vi "CRYASIO Receive Global Data.vi"(8 "buf count":i32=-1, 9 "Chn Idx":u32, 10 "Data Length":i32, 11 "Last Remain Buffer":i32[](array[numeric])) -> (0 "Over Load":i32, 1 "bufCount":i32, 2 "Data Out":i32[](array[numeric]), 3 "Remain Data":i32[](array[numeric]))   [LabVIEW 2013]
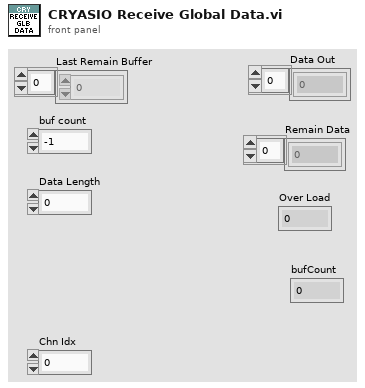
[diagram p1: front panel]
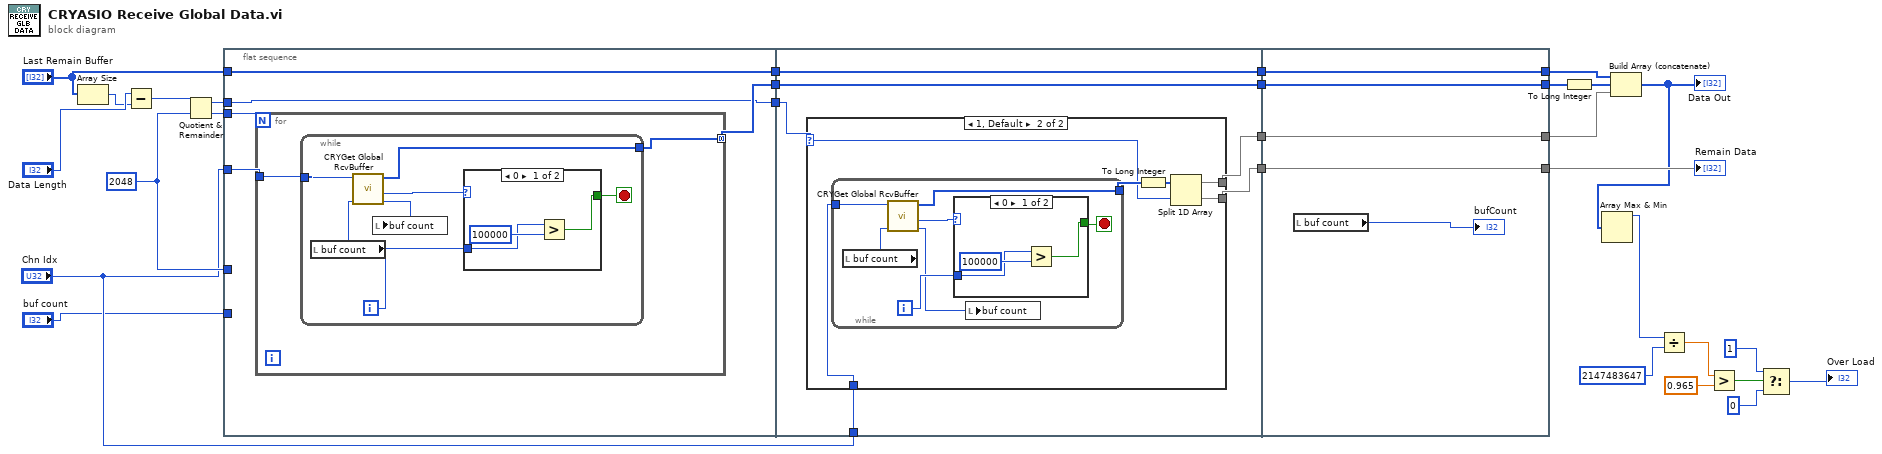
[diagram p0: block diagram]
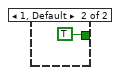
[diagram p2: hidden frame]
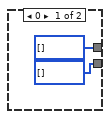
[diagram p3: hidden frame]
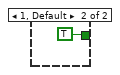
[diagram p4: hidden frame]
diagram:
  w30 = 2048 ("y")
  n1 = Array Size(array="Last Remain Buffer") -> (size(s)=w28:i32)
  n2 = Subtract(x="Data Length", y=w28) -> (x-y=w27:i32)
  n3 = Quotient & Remainder(x=w27, y=w30) -> (x-y*floor(x/y)=w19:i32, floor(x/y)=w26:i32)
  n4 = flat-sequence {
    tunnel: w30 -> [_]
    tunnel: w26 -> [w35]
    tunnel: [w34] -> w23
    tunnel: [w33] -> w22
    tunnel: "Last Remain Buffer" -> [w33]
    tunnel: w19 -> [w32]
    tunnel: [w32] -> w18
    tunnel: "Chn Idx" -> [w31]
    tunnel: "buf count" -> [_]
    tunnel: w23 -> [w54]
    tunnel: w22 -> [w53]
    tunnel: w18 -> [w52]
    tunnel: "Chn Idx" -> [w49]
    tunnel: [w54] -> w13
    tunnel: [w53] -> w12
    tunnel: [w51] -> w11
    tunnel: [w50] -> w10
    tunnel: [w75] -> w16
    tunnel: [w76] -> w17
    tunnel: [w77] -> w20
    tunnel: [w78] -> w25
    tunnel: w13 -> [w78]
    tunnel: w12 -> [w77]
    tunnel: w11 -> [w76]
    tunnel: w10 -> [w75]
    frame #0 {
      n5 = for {
        N: w35 -> [_]
        tunnel: [w37] -> w34 mode=concatenating
        tunnel: w31 -> [w36]
        n6 = while {
          tunnel: [w42] -> w37
          tunnel: w36 -> [w41]
          i -> [w40]
          stop <- w43 stop-if-true
          n7 = local read "buf count"() -> (w38:i32)
          n8 = call "CRYGet Global RcvBuffer.vi"("bufCount In"=w38, "Chn Idx"=w41) -> ("bufCount"=w39:i32, "rtn value"=w44:i32, "Data"=w42:i32[])  [unwired: 5 in]
          n9 = local write "buf count"(w39) -> ()
          n10 = case shown="0" w44 {
            tunnel: [w46 TRUE] -> w43
            tunnel: w40 -> [w45 _]
            frame 0 {
              n11 = Greater?(x=w45, y=100000) -> (0:w46:bool)
            }
            frame 1, Default {
            }
          }
        }
      }
    }
    frame #1 {
      n12 = case shown="1, Default" w52 {
        selector: w52 -> [_ w57]
        tunnel: [i32[] [] w61] -> w51
        tunnel: [i32[] [] w60] -> w50
        tunnel: w49 -> [_ w58]
        frame 0 {
        }
        frame 1, Default {
          n13 = while {
            tunnel: [w67] -> w62
            tunnel: w58 -> [w66]
            i -> [w65]
            stop <- w68 stop-if-true
            n14 = local read "buf count"() -> (w64:i32)
            n15 = call "CRYGet Global RcvBuffer.vi"("bufCount In"=w64, "Chn Idx"=w66) -> ("bufCount"=w63:i32, "rtn value"=w69:i32, "Data"=w67:i32[])  [unwired: 5 in]
            n16 = case shown="0" w69 {
              tunnel: [w71 TRUE] -> w68
              tunnel: w65 -> [w70 _]
              frame 0 {
                n17 = Greater?(x=w70, y=100000) -> (0:w71:bool)
              }
              frame 1, Default {
              }
            }
            n18 = local write "buf count"(w63) -> ()
          }
          n19 = To Long Integer(number=w62) -> (32bit integer=w59:i32[])
          n20 = Split 1D Array(array=w59, index=w57) -> (first subarray=w61:i32[], second subarray=w60:i32[])
        }
      }
    }
    frame #2 {
      n21 = local read "buf count"() -> (→"bufCount":i32)
    }
  }
  n22 = To Long Integer(number=w25) -> (32bit integer=w24:i32[])
  n23 = Build Array (concatenate)(w20, w24, w17) -> (w1:i32[])
  "Data Out" <- w1
  n24 = Array Max & Min(array=w1) -> (max value=w7:i32)  [unwired: 3 out]
  n25 = Divide(x=w7, y=2147483647) -> (x/y=w8:dbl)
  n26 = Greater?(x=w8, y=0.965) -> (0:w3:bool)
  n27 = Select(t=1 ("y"), s=w3, f=0 ("y")) -> (s? t:f=→"Over Load":i32)
  "Remain Data" <- w16
